vi "Get Property.vi"(10 "Ctl Ref":refnum<vi>, 11 "UIP In":refnum<class "DescriptionUIP.lvclass">) -> (0 "Error Out":errorcluster, 3 "UIP Out":refnum<class "DescriptionUIP.lvclass">)   [LabVIEW 2015, in "DescriptionUIP.lvclass"]
doc: "Modify this method to implement functionality for extracting the property from VI Server Control to be stored inside UIP."
uses:
  DescriptionUIP.lvclass
  DescriptionUIP.lvclass/DescriptionUIP.ctl
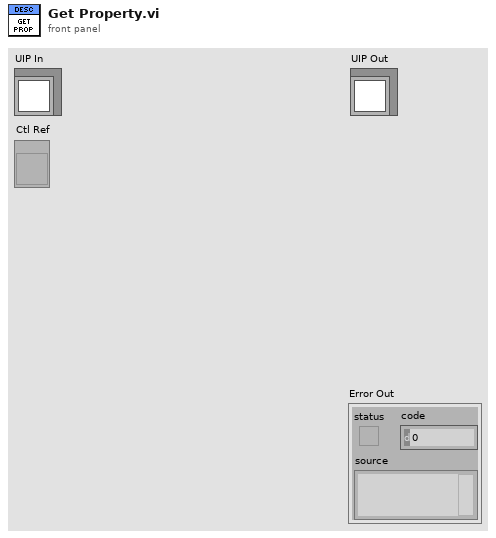
[diagram p1: front panel]
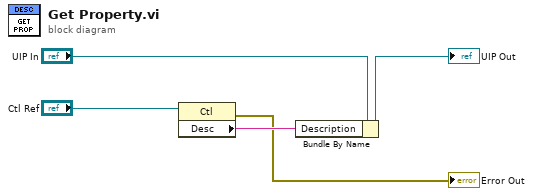
[diagram p0: block diagram]
diagram:
  n1 = property class="Ctl"(reference="Ctl Ref") -> (error out=→"Error Out":errorcluster, "Desc"=w2:string)  [unwired: 1 in, 1 out]
  n2 = Bundle By Name(cluster="UIP In", "Description"=w2) -> (→"UIP Out":refnum<class "DescriptionUIP.lvclass">)
